vi "Smoothing.vi"(7 "Warming up?":bool, 10 "Number to Average":i32=30, 11 "O2%":dbl format="%#_13g") -> (3 "Mean O2%":dbl)   [LabVIEW 2013]
uses:
  <vilib>/ptbypt/NI_PtbyPt.lvlib
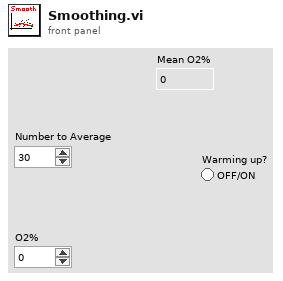
[diagram p1: front panel]
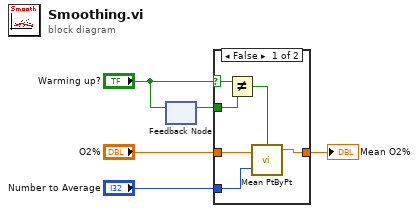
[diagram p0: block diagram]
diagram:
  n1 = feedback-in #1("Warming up?") -> ()
  n2 = feedback #1() -> (w2:bool)  [unwired: 1 in]
  n3 = case shown="False" "Warming up?" {
    selector: "Warming up?" -> [w9 _]
    tunnel: "O2%" -> [w11 w12]
    tunnel: "Number to Average" -> [w10 _]
    tunnel: w2 -> [w8 _]
    tunnel: [w7 w12] -> w1
    frame False {
      n4 = Not Equal?(x=w9, y=w8) -> (x != y?=w6:bool)
      n5 = call <vilib>:"Mean PtByPt.vi"("x"=w11, "sample length"=w10, "initialize"=w6) -> ("mean"=w7:dbl)  [unwired: 1 in, 1 out]
    }
    frame True {
    }
  }
  "Mean O2%" <- w1
